vi "读取物种名.vi"(8 "error in (no error)":errorcluster caption="错误输入（无错误）", 11 "Animal输入":refnum<class "Animal.lvclass">) -> (0 "error out":errorcluster caption="错误输出", 2 "物种名":string, 3 "Animal输出":refnum<class "Animal.lvclass">)   [LabVIEW 2020, in "Animal.lvclass"]
uses:
  Animal.lvclass
  Animal.lvclass/Animal.ctl
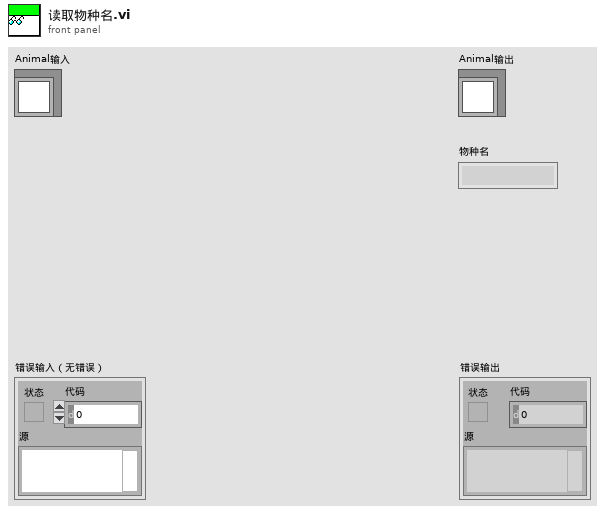
[diagram p1: front panel]
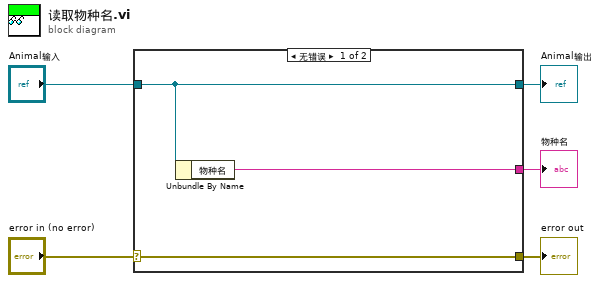
[diagram p0: block diagram]
diagram:
  n1 = case shown="无错误" "error in (no error)" {
    selector: "error in (no error)" -> [w8 w9]
    tunnel: [w8 w9] -> w4
    tunnel: [w7 w10] -> w2
    tunnel: "Animal输入" -> [w7 w10]
    tunnel: [w6 _] -> w1
    frame No Error {
      n2 = Unbundle By Name(w7) -> ("物种名"=w6:string)
    }
    frame Error {
    }
  }
  "error out" <- w4
  "Animal输出" <- w2
  "物种名" <- w1
